vi "LaserCal-Process Data (Dynamic).vi"(7 "Power (W)":dbl, 9 "I-O Data in":T1, 11 "error in (no error)":errorcluster, 12 "Seq Index":i32) -> (10 "I-O Data out":T1, 15 "error out":errorcluster)   [LabVIEW 2015]
uses:
  Typedefs/LaserCal-Data (Dynamic).ctl
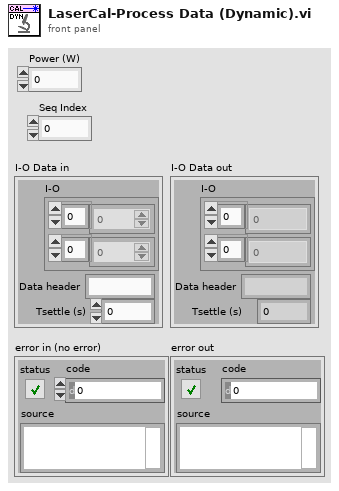
[diagram p1: front panel]
types:
  T1 = typedef "LaserCal-Data (Dynamic).ctl" = cluster{"I-O":cluster{dbl[], dbl[]}, "Data header":string, "Tsettle (s)":dbl}
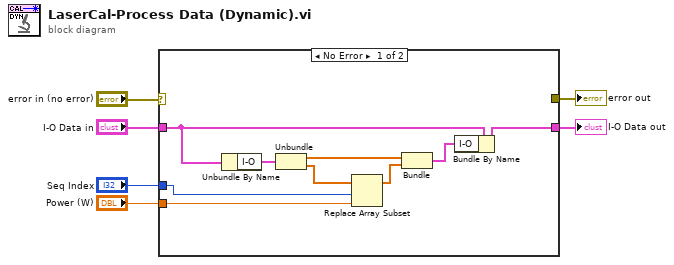
[diagram p0: block diagram]
diagram:
  n1 = case shown="No Error" "error in (no error)" {
    selector: "error in (no error)" -> [_ w17]
    tunnel: [_ w17] -> w2
    tunnel: "I-O Data in" -> [w15 w16]
    tunnel: [w11 w16] -> w4
    tunnel: "Seq Index" -> [w10 _]
    tunnel: "Power (W)" -> [w14 _]
    frame No Error {
      n2 = Unbundle By Name(w15) -> ("I-O"=w8:cluster{dbl[], dbl[]})
      n3 = Unbundle(w8) -> (w9:dbl[], w13:dbl[])
      n4 = Replace Array Subset(array=w13, new element=w14, index=w10) -> (w12:dbl[])
      n5 = Bundle(w9, w12) -> (w7:cluster{dbl[], dbl[]})  [unwired: 1 in]
      n6 = Bundle By Name(cluster=w15, "I-O"=w7) -> (w11:T1)
    }
    frame Error {
    }
  }
  "I-O Data out" <- w4
  "error out" <- w2
